vi "In Place Read 1D Array I32.vi"(8 "error in (no error)":errorcluster, 9 "start index (0)":i64, 10 "values in":i32[](array[numeric]), 11 "pointer in":u64) -> (0 "error out":errorcluster, 1 "start index out":i64, 2 "values out":i32[](array[numeric]), 3 "pointer out":u64)   [LabVIEW 2013, in "Linux RT IPC.Shared Memory.lvlib"]
uses:
  Linux RT IPC.Shared Memory.lvlib
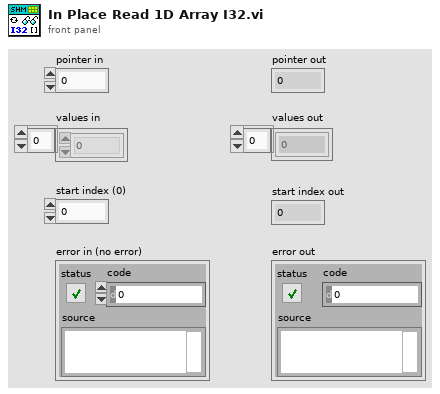
[diagram p1: front panel]
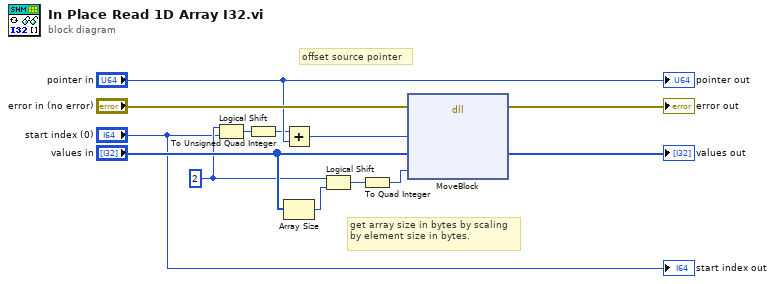
[diagram p0: block diagram]
diagram:
  w4 = i16 2 ("y")
  # "get array size in bytes by scaling by element size in bytes."
  # "offset source pointer"
  n1 = Logical Shift(y=w4, x="start index (0)") -> (x << y=w7:i64)
  n2 = To Unsigned Quad Integer(1:w7) -> (0:w3:u64)
  n3 = Add(x=w3, y="pointer in") -> (x+y=w5:u64)
  n4 = Array Size(array="values in") -> (size(s)=w2:i32)
  n5 = Logical Shift(y=w4, x=w2) -> (x << y=w8:i32)
  n6 = To Quad Integer(1:w8) -> (0:w6:i64)
  n7 = dll-call lib="LabVIEW" fn="MoveBlock"(error in="error in (no error)", "pointer"=w5, "data"="values in", "size"=w6) -> (error out=→"error out":errorcluster, "data"=→"values out":i32[])  [unwired: 5 in, 1 out]
  "pointer out" <- "pointer in"
  "start index out" <- "start index (0)"
